vi "Histogram Main.vi"() -> ()   [LabVIEW 2012]
uses:
  Consumer Message.ctl
panel:
  out "波形图表":dbl[](graph)
  in  "快照":bool
  out "直方图":cluster{"histogram":dbl[], "x axis":dbl[]}(graph)
  out "消费者关闭？":bool
  in  "停止":bool
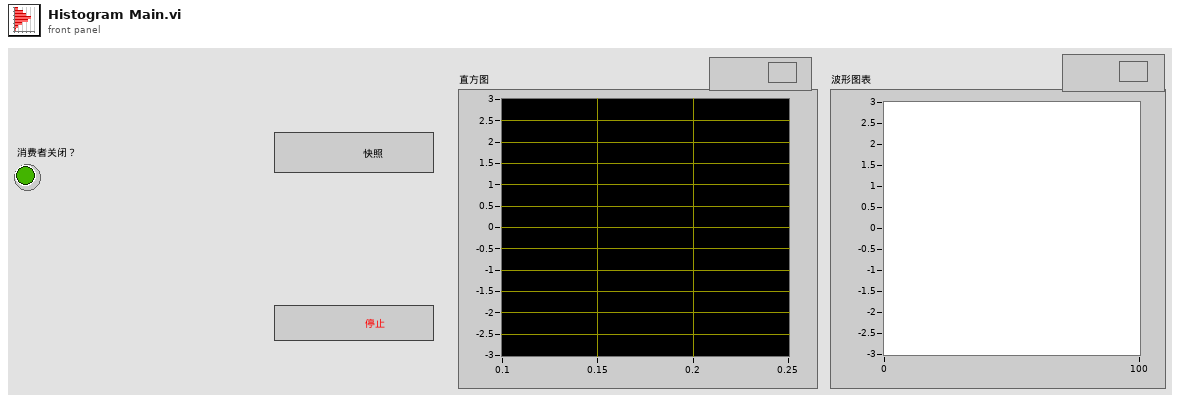
[diagram p1: front panel]
types:
  T1 = typedef "Consumer Message.ctl" = cluster{"消费者状态":string, "布尔数据":bool, "数值数据":i32, "信号":dbl[], "错误":cluster{"状态":bool, "代码":i32, "源":string}}
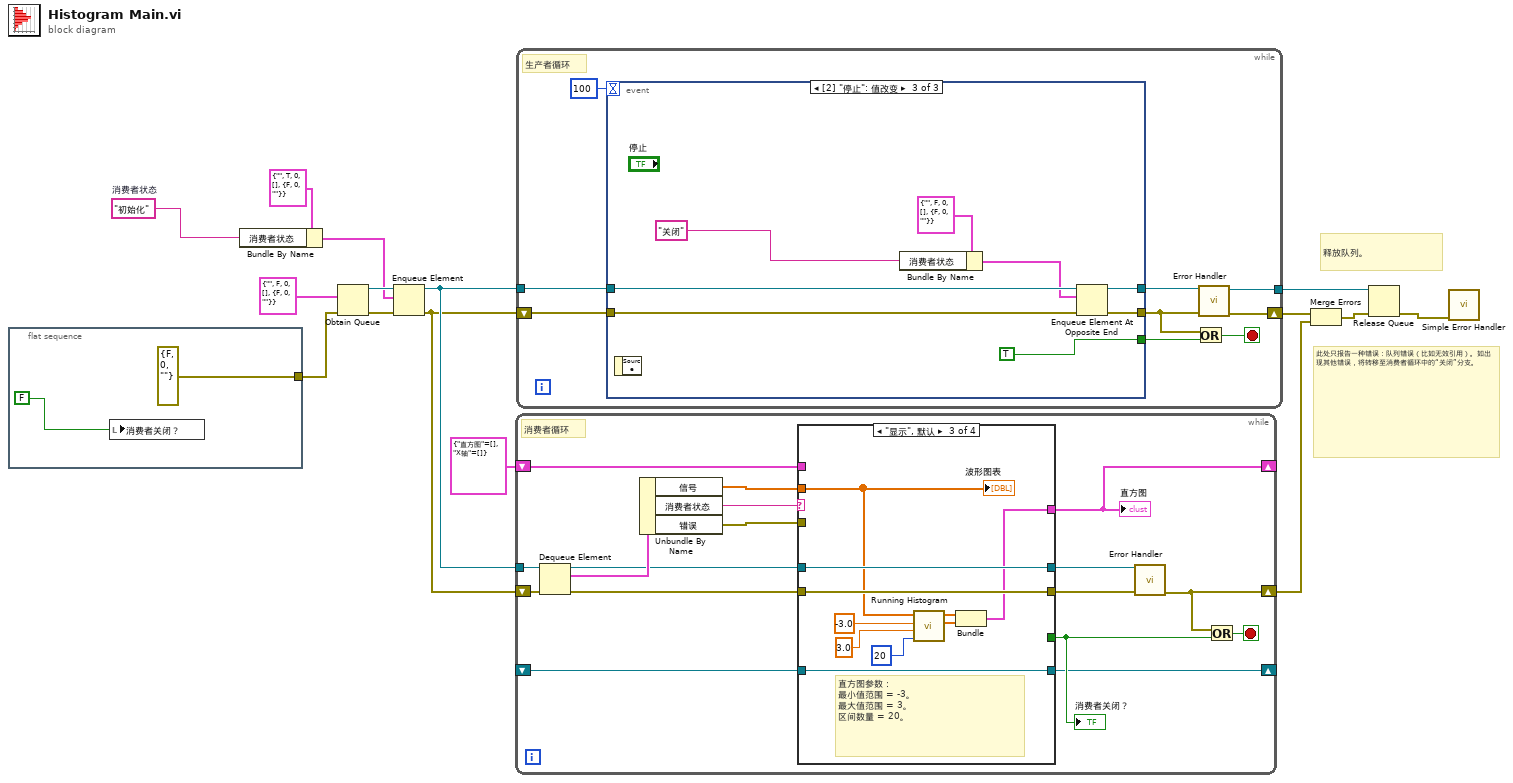
[diagram p0: block diagram]
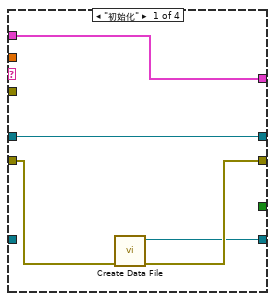
[diagram p2: hidden frame]
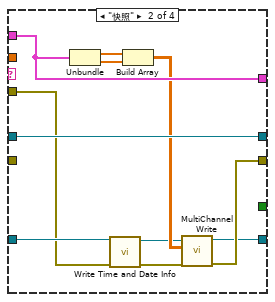
[diagram p3: hidden frame]
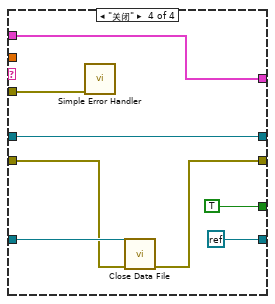
[diagram p4: hidden frame]
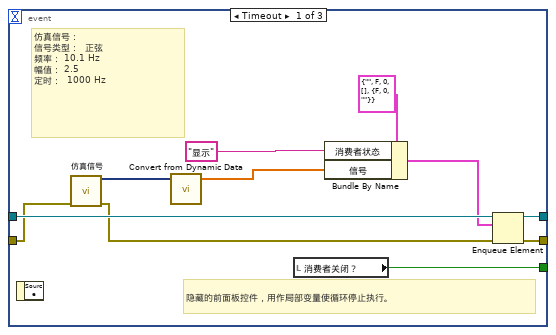
[diagram p5: hidden frame]
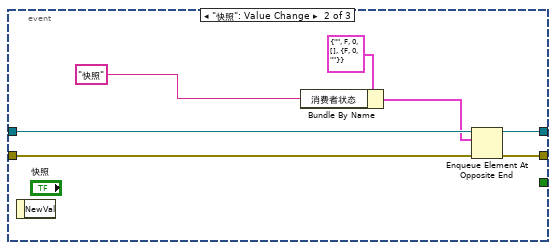
[diagram p6: hidden frame]
diagram:
  w8 = "初始化"  # 消费者状态
  # "释放队列。"
  # "此处只报告一种错误：队列错误（比如无效引用）。如出现其他错误，将转移至消费者循环中的“关闭”分支。"
  n1 = flat-sequence {
    tunnel: [cluster{"状态":bool, "代码":i32, "源":string} {"状态"=FALSE, "代码"=0, "源"=""} ("错误输入（无错误）")] -> w11
    frame #0 {
      n2 = local write "消费者关闭？"(FALSE ("停止循环（局部）")) -> ()
    }
  }
  n3 = Bundle By Name ("按名称捆绑")(cluster=T1 {"消费者状态"="", "布尔数据"=TRUE, "数值数据"=0, "信号"=[], "错误"={"状态"=FALSE, "代码"=0, "源"=""}} ("消费者消息"), "消费者状态"=w8) -> (w9:T1)
  n4 = Obtain Queue ("获取队列引用")(element data type=T1 {"消费者状态"="", "布尔数据"=FALSE, "数值数据"=0, "信号"=[], "错误"={"状态"=FALSE, "代码"=0, "源"=""}}, error in (no error)=w11) -> (queue out=w13:refnum<queue>, error out=w15:errorcluster)  [unwired: 3 in, 1 out]
  n5 = Enqueue Element ("元素入队列")(queue=w13, element=w9, error in (no error)=w15) -> (queue out=w12:refnum<queue>, error out=w2:errorcluster)  [unwired: 1 in, 1 out]
  n6 = while {
    tunnel: w12 -> [w34]
    shift-right: [w25] -> w6
    shift-left: w2 -> [w33]
    shift-right: [w18] -> _
    shift-left: cluster{"直方图":dbl[], "X轴":dbl[]} {"直方图"=[], "X轴"=[]} -> [w22]
    shift-right: [w19] -> _
    shift-left: _ -> [w20]
    stop <- w26 stop-if-true
    # "消费者循环"
    n7 = Dequeue Element ("元素出队列")(queue=w34, error in (no error)=w33) -> (queue out=w24:refnum<queue>, element=w32:T1, error out=w23:errorcluster)  [unwired: 1 in, 1 out]
    n8 = Unbundle By Name ("按名称解除捆绑")(w32) -> ("信号"=w21:dbl[], "消费者状态"=w31:string, "错误"=w28:cluster{"状态":bool, "代码":i32, "源":string})
    n9 = case shown="\"显示\", 默认" w31 {
      tunnel: [_ _ _ TRUE] -> w27
      tunnel: w23 -> [w37 _ w59 w63]
      tunnel: [w36 w46 w59 w62] -> w30
      tunnel: w24 -> [w39 w50 w60 w66]
      tunnel: [w39 w50 w60 w66] -> w29
      tunnel: w28 -> [_ w40 _ w67]
      tunnel: [w38 w48 w56 w65] -> w18
      tunnel: w22 -> [w38 w48 _ w65]
      tunnel: w21 -> [_ _ w54 _]
      tunnel: w20 -> [_ w41 w55 w64]
      tunnel: [w35 w45 w55 refnum<k0> refnum ("非法引用句柄常量")] -> w19
      frame "初始化" {
        n10 = call "Create Data File.vi"("错误输入"=w37) -> ("错误输出"=w36:cluster{"状态":bool, "代码":i32, "源":string}, "文件引用句柄"=w35:refnum<file>)  [unwired: 9 in]
      }
      frame "快照" {
        n11 = Unbundle ("解除捆绑")(w48) -> ("直方图"=w44:dbl[], "X轴"=w49:dbl[])
        n12 = call "Write Time and Date Info.vi"("错误输入"=w40, "文件引用句柄输入"=w41) -> ("错误输出"=w42:cluster{"状态":bool, "代码":i32, "源":string}, "文件引用句柄输出"=w43:refnum<file>)  [unwired: 6 in]
        n13 = Build Array ("创建数组")(w44, w49) -> (w47:dbl[][])
        n14 = call "MultiChannel Write.vi"("错误输入"=w42, "数据至记录"=w47, "文件引用句柄输入"=w43) -> ("错误输出"=w46:cluster{"状态":bool, "代码":i32, "源":string}, "文件引用句柄输出"=w45:refnum<file>)  [unwired: 7 in]
      }
      frame "显示", Default {
        # "直方图参数：\n最小值范围 = -3。\n最大值范围 = 3。\n区间数量 = 20。"
        n15 = call "Running Histogram.vi"("区间"=20, "最大值"=3.0, "最小值"=-3.0, "输入数据"=w54) -> ("X轴"=w57:dbl[], "直方图"=w58:dbl[])  [unwired: 4 in, 2 out]
        n16 = Bundle ("捆绑")("直方图"=w58, "X轴"=w57) -> (w56:cluster{"直方图":dbl[], "X轴":dbl[]})  [unwired: 1 in]
        "波形图表" <- w54
      }
      frame "关闭" {
        n17 = call <vilib>:"Simple Error Handler.vi"("error in (no error)"=w67) -> ()  [unwired: 4 in, 5 out]
        n18 = call "Close Data File.vi"("错误输入"=w63, "文件引用句柄输入"=w64) -> ("错误输出"=w62:errorcluster)  [unwired: 9 in]
      }
    }
    "消费者关闭？" <- w27
    "直方图" <- w18
    n19 = call "Error Handler.vi"("错误输入"=w30, "队列输入"=w29) -> ("错误输出"=w25:cluster{"状态":bool, "代码":i32, "源":string})  [unwired: 8 in, 1 out]
    n20 = Or ("或")(x=w25, y=w27) -> (x .or. y?=w26:bool)
  }
  n21 = while {
    tunnel: w12 -> [w77]
    shift-right: [w70] -> w7
    shift-left: w2 -> [w76]
    tunnel: [w69] -> w1
    stop <- w72 stop-if-true
    # "生产者循环"
    n22 = event shown="[2] \"停止\": 值改变" {
      selector: _ -> [_ _ _]
      dyn-events: _ -> [_ _ _]
      timeout: 100 -> [_ _ _]
      tunnel: w77 -> [w87 w94 w103]
      tunnel: w76 -> [w80 w93 w101]
      tunnel: [w82 w95 w100] -> w71
      tunnel: [w88 _ TRUE] -> w73
      tunnel: [w83 w90 w99] -> w75
      event Timeout {
        # "仿真信号：\n信号类型：  正弦\n频率： 10.1 Hz\n幅值： 2.5\n定时：  1000 Hz"
        # "隐藏的前面板控件，用作局部变量使循环停止执行。"
        n23 = event-data ("事件数据节点")() -> ()  [unwired: 1 in, 1 out]
        n24 = call "仿真信号"("error in (no error)"=w80) -> ("正弦与均匀噪声"=w78:dynamicdata, "error out"=w79:errorcluster)  [unwired: 13 in]
        n25 = call "Convert from Dynamic Data"("Dynamic Data Type"=w78) -> ("Array"=w81:dbl[])  [unwired: 3 in]
        n26 = local read "消费者关闭？"() -> (w88:bool)
        n27 = Bundle By Name ("按名称捆绑")(cluster=T1 {"消费者状态"="", "布尔数据"=FALSE, "数值数据"=0, "信号"=[], "错误"={"状态"=FALSE, "代码"=0, "源"=""}}, "消费者状态"="显示", "信号"=w81) -> (w85:T1)
        n28 = Enqueue Element ("元素入队列")(queue=w87, element=w85, error in (no error)=w79) -> (queue out=w83:refnum<queue>, error out=w82:errorcluster)  [unwired: 1 in, 1 out]
      }
      event "快照": Value Change {
        n29 = event-data ("事件数据节点")() -> ()  [unwired: 1 in, 1 out]
        n30 = Bundle By Name ("按名称捆绑")(cluster=T1 {"消费者状态"="", "布尔数据"=FALSE, "数值数据"=0, "信号"=[], "错误"={"状态"=FALSE, "代码"=0, "源"=""}}, "消费者状态"="快照" ("字符串数据")) -> (w91:T1)
        n31 = Enqueue Element At Opposite End ("队列最前端插入元素")(queue=w94, element=w91, error in (no error)=w93) -> (queue out=w90:refnum<queue>, error out=w95:errorcluster)  [unwired: 1 in, 1 out]
      }
      event "停止": Value Change {
        n32 = event-data ("事件数据节点")() -> ()  [unwired: 1 in, 1 out]
        n33 = Bundle By Name ("按名称捆绑")(cluster=T1 {"消费者状态"="", "布尔数据"=FALSE, "数值数据"=0, "信号"=[], "错误"={"状态"=FALSE, "代码"=0, "源"=""}}, "消费者状态"="关闭") -> (w96:T1)
        n34 = Enqueue Element At Opposite End ("队列最前端插入元素")(queue=w103, element=w96, error in (no error)=w101) -> (queue out=w99:refnum<queue>, error out=w100:errorcluster)  [unwired: 1 in, 1 out]
      }
    }
    n35 = Or ("或")(x=w71, y=w73) -> (x .or. y?=w72:bool)
    n36 = call "Error Handler.vi"("错误输入"=w71, "队列输入"=w75) -> ("错误输出"=w70:cluster{"状态":bool, "代码":i32, "源":string}, "队列输出"=w69:refnum<queue>)  [unwired: 8 in]
  }
  n37 = Merge Errors ("合并错误")(w7, w6) -> (w4:errorcluster)
  n38 = Release Queue ("释放队列引用")(queue=w1, error in (no error)=w4) -> (error out=w3:errorcluster)  [unwired: 1 in, 2 out]
  n39 = call <vilib>:"Simple Error Handler.vi"("error in (no error)"=w3) -> ()  [unwired: 4 in, 5 out]
